vi "get_nofPersons.vi"(0 "MySociety":refnum<class "HB_Society.lvclass">, 5 "error in (no error)":errorcluster) -> (14 "dup MySociety":refnum<class "HB_Society.lvclass">, 16 "nofPersons":dbl, 19 "error out":errorcluster)   [LabVIEW 2009, in "HB_BaseClass_Examples.lvlib" / "HB_Society.lvclass"]
doc: "Returns the sum of nofPersons of THIS object."
uses:
  HB_Society.lvclass
  HB_Society.lvclass/HB_Society.ctl
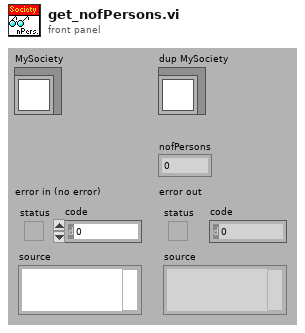
[diagram p1: front panel]
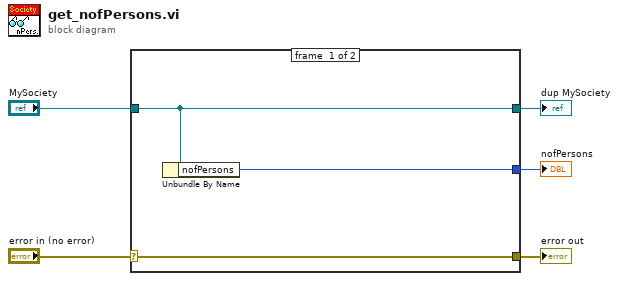
[diagram p0: block diagram]
diagram:
  n1 = case shown="No Error" "error in (no error)" {
    selector: "error in (no error)" -> [w8 w9]
    tunnel: [w8 w9] -> w4
    tunnel: [w7 w10] -> w2
    tunnel: "MySociety" -> [w7 w10]
    tunnel: [w6 _] -> w1
    frame #0 {
      n2 = Unbundle By Name(w7) -> ("nofPersons"=w6:i32)
    }
    frame #1 {
    }
  }
  "error out" <- w4
  "dup MySociety" <- w2
  "nofPersons" <- w1
